vi "Count_Test_load.vi"(0 "tsd":sgl[](array[numeric]), 1 "Test":sgl[][](array[numeric])) -> (2 "dev":sgl[](array[numeric]) format="%#.2g", 3 "devs":string[](array[string]), 4 "inacc":sgl[](array[numeric]) format="%#.2g", 5 "inaccs":string[](array[string]))   [LabVIEW 2019]
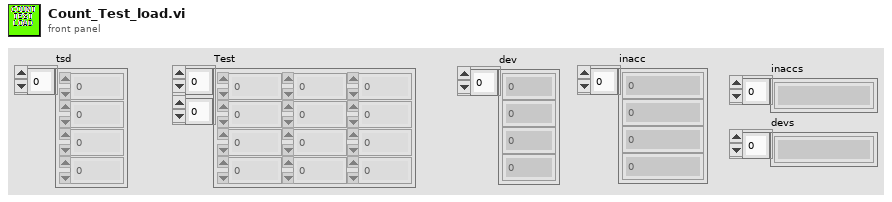
[diagram p1: front panel]
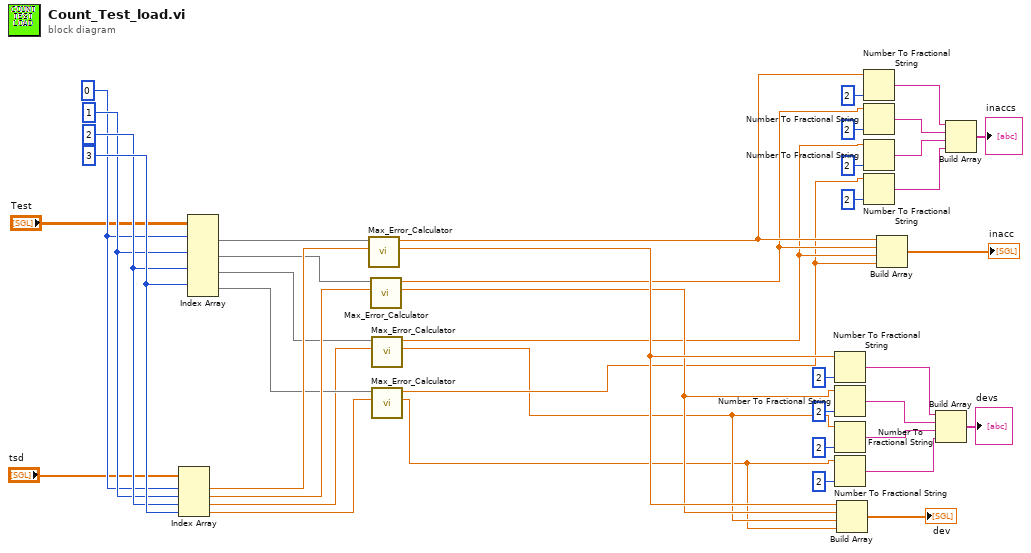
[diagram p0: block diagram]
diagram:
  w42 = 3 ("索引 (行)")
  w41 = 2 ("索引 (行)")
  w40 = 1 ("索引 (行)")
  w39 = 0 ("索引 (行)")
  n1 = Index Array(array="tsd", index #1=w39, index #2=w40, index #3=w41, index #4=w42) -> (element #1=w17:sgl, element #2=w13:sgl, element #3=w8:sgl, element #4=w7:sgl)
  n2 = Index Array(array="Test", index (row) #1=w39, index (row) #2=w40, index (row) #3=w41, index (row) #4=w42) -> (element #1=w18:sgl[], element #2=w14:sgl[], element #3=w10:sgl[], element #4=w9:sgl[])  [unwired: 4 in]
  n3 = call "Max_Error_Calculator.vi"("数值"=w17, "数组"=w18) -> ("dev"=w15:sgl, "inaccc"=w16:sgl)  [unwired: 8 in]
  n4 = call "Max_Error_Calculator.vi"("数值"=w13, "数组"=w14) -> ("dev"=w11:sgl, "inaccc"=w12:sgl)  [unwired: 8 in]
  n5 = call "Max_Error_Calculator.vi"("数值"=w8, "数组"=w10) -> ("dev"=w4:sgl, "inaccc"=w6:sgl)  [unwired: 8 in]
  n6 = call "Max_Error_Calculator.vi"("数值"=w7, "数组"=w9) -> ("dev"=w3:sgl, "inaccc"=w5:sgl)  [unwired: 8 in]
  n7 = Number To Fractional String(number=w15, precision (6)=i16 2 ("精度(6)")) -> (F-format string=w23:string)  [unwired: 2 in]
  n8 = Number To Fractional String(number=w11, precision (6)=i16 2 ("精度(6)")) -> (F-format string=w22:string)  [unwired: 2 in]
  n9 = Number To Fractional String(number=w4, precision (6)=i16 2 ("精度(6)")) -> (F-format string=w21:string)  [unwired: 2 in]
  n10 = Number To Fractional String(number=w3, precision (6)=i16 2 ("精度(6)")) -> (F-format string=w20:string)  [unwired: 2 in]
  n11 = Build Array(w15, w11, w4, w3) -> (→"dev":sgl[])
  n12 = Number To Fractional String(number=w16, precision (6)=i16 2 ("精度(6)")) -> (F-format string=w28:string)  [unwired: 2 in]
  n13 = Number To Fractional String(number=w12, precision (6)=i16 2 ("精度(6)")) -> (F-format string=w27:string)  [unwired: 2 in]
  n14 = Number To Fractional String(number=w6, precision (6)=i16 2 ("精度(6)")) -> (F-format string=w26:string)  [unwired: 2 in]
  n15 = Number To Fractional String(number=w5, precision (6)=i16 2 ("精度(6)")) -> (F-format string=w25:string)  [unwired: 2 in]
  n16 = Build Array(w16, w12, w6, w5) -> (→"inacc":sgl[])
  n17 = Build Array(w23, w22, w21, w20) -> (→"devs":string[])
  n18 = Build Array(w28, w27, w26, w25) -> (→"inaccs":string[])
